vi "get 1d spectrum data.vi"(6 "data in":T1={"Total counts"=0, "cps"=0.0, "live time"=0.0, "pulser"=0.0, "rare counts"=0.0, "other counts"=0.0, "total run time(sec)"=0.0, "adjusted run time(sec)"=0.0, "17O average"=1.0, "17O current"=1.0}, 8 "error in":errorcluster, 9 "gates":i32[](array[numeric]), 10 "time in":u32) -> (0 "error out 2":errorcluster, 1 "MCAHistograms":u32[](array[numeric]), 2 "data out":T1={"Total counts"=0, "cps"=0.0, "live time"=0.0, "pulser"=0.0, "rare counts"=0.0, "other counts"=0.0, "total run time(sec)"=0.0, "adjusted run time(sec)"=0.0, "17O average"=1.0, "17O current"=1.0}, 3 "MCA Histograms":u32[](graph), 4 "pulser events":dbl format="%0.2f")   [LabVIEW 2016]
doc: "gathers 1d spectrum data for further analysis"
uses:
  controls/count control.ctl
  <vilib>/DAQmx/read.llb/DAQmx Read (Counter DBL 1Chan 1Samp).vi
  <vilib>/DAQmx/miscellaneous.llb/DAQmx Fill In Error Info.vi
  Drivers/Pixie4DLL.dll
panel:
  out "error out":errorcluster
  out "adjusted run time":dbl
  out "total run time":dbl
  out "live time":dbl
  out "cps":dbl
  out "counts":u32
  out "pulser":dbl format="%0.2f"
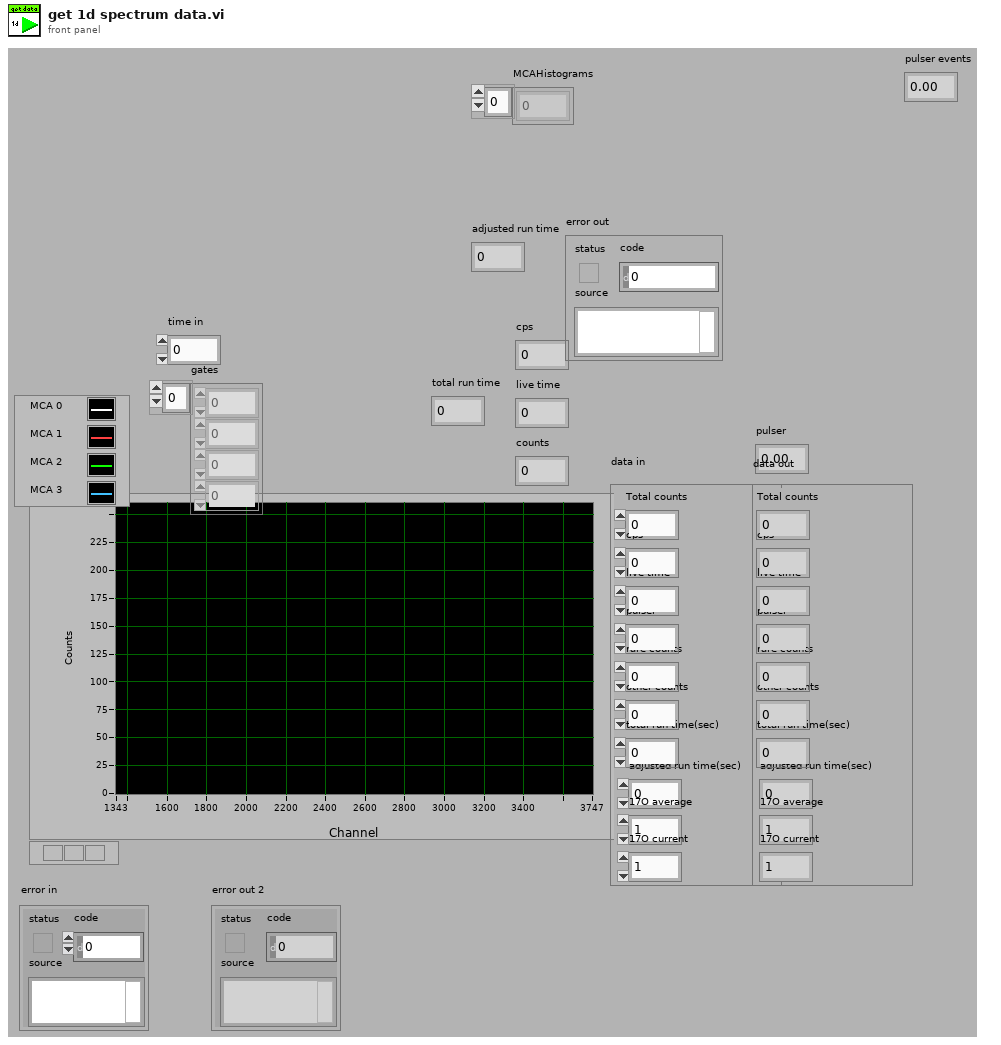
[diagram p1: front panel]
types:
  T1 = typedef "count control.ctl" = cluster{"Total counts":u32, "cps":dbl, "live time":dbl, "pulser":dbl, "rare counts":dbl, "other counts":dbl, "total run time(sec)":dbl, "adjusted run time(sec)":dbl, "17O average":dbl, "17O current":dbl}
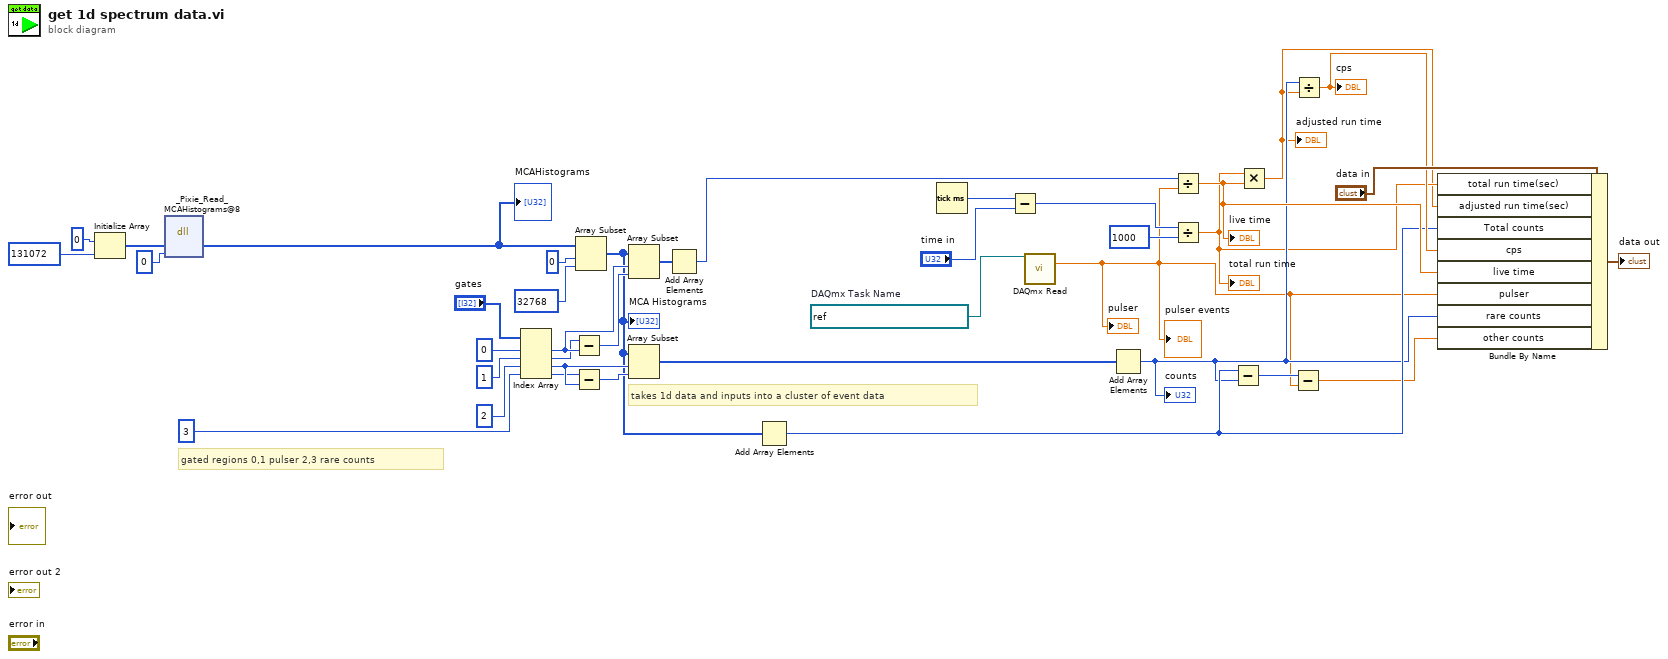
[diagram p0: block diagram]
diagram:
  w3 = refnum<k21> "MyCountEdgesTask"  # DAQmx Task Name
  # "takes 1d data and inputs into a cluster of event data"
  # "gated regions 0,1 pulser 2,3 rare counts"
  n1 = Initialize Array(0, 131072) -> (w17:i32[])
  n2 = dll-call lib="D:/Users/wymanm/Desktop/DAQuiri - 2017a/lois/Drivers/Pixie4DLL.dll" fn="_Pixie_Read_MCAHistograms@8"("MCAHistograms"=w17, "ModNum"=u16 0 ("Module number")) -> ("MCAHistograms"=w15:u32[])  [unwired: 5 in, 2 out]
  "MCAHistograms" <- w15
  n3 = Index Array(array="gates", index #1=0 ("index"), index #2=1 ("index"), index #3=2 ("index"), index #4=3 ("index")) -> (element #1=w32:i32, element #2=w31:i32, element #3=w36:i32, element #4=w35:i32)
  n4 = Subtract(x=w31, y=w32) -> (x-y=w33:i32)
  n5 = Subtract(x=w35, y=w36) -> (x-y=w34:i32)
  n6 = Array Subset(array=w15, index=0, length=32768) -> (w11:u32[])
  "MCA Histograms" <- w11
  n7 = Array Subset(array=w11, index=w32, length=w33) -> (w38:u32[])
  n8 = Array Subset(array=w11, index=w36, length=w34) -> (w37:u32[])
  n9 = Add Array Elements(numeric array=w38) -> (sum=w2:u32)
  n10 = Add Array Elements(numeric array=w11) -> (sum=w10:u32)
  n11 = Tick Count (ms)() -> (millisecond timer value=w22:u32)
  n12 = Subtract(x=w22, y="time in") -> (x-y=w24:u32)
  n13 = call-poly <vilib>:"DAQmx Read.vi"("task/channels in"=w3) -> ("data"=w1:dbl)  [unwired: 12 in, 2 out]
  "pulser" <- w1
  "pulser events" <- w1
  n14 = Add Array Elements(numeric array=w37) -> (sum=w9:u32)
  "counts" <- w9
  n15 = Divide(x=w2, y=w1) -> (x/y=w13:dbl)
  "live time" <- w13
  n16 = Divide(x=w24, y=u32 1000) -> (x/y=w6:dbl)
  "total run time" <- w6
  n17 = Subtract(x=w10, y=w9) -> (x-y=w8:u32)
  n18 = Multiply(x=w6, y=w13) -> (x*y=w5:dbl)
  "adjusted run time" <- w5
  n19 = Subtract(x=w8, y=w1) -> (x-y=w7:dbl)
  n20 = Divide(x=w9, y=w5) -> (x/y=w12:dbl)
  "cps" <- w12
  n21 = Bundle By Name(cluster="data in", "total run time(sec)"=w6, "adjusted run time(sec)"=w5, "Total counts"=w10, "cps"=w12, "live time"=w13, "pulser"=w1, "rare counts"=w9, "other counts"=w7) -> (→"data out":T1)
